vi "Tips.vi"() -> ()   [LabVIEW 2022 SP3]
panel:
  out "Numeric":i32
  out "x+y":dbl
  in  "y":dbl
  in  "x":dbl
  # "Ctrl + B 删除断线\nCtrl + R 运行程序\nCtrl+ E  更换面板"
  # "This is commit!"
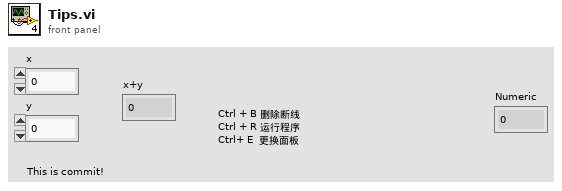
[diagram p1: front panel]
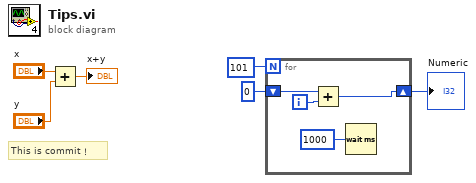
[diagram p0: block diagram]
diagram:
  # "This is commit！"
  n1 = Add(x="x", y="y") -> (x+y=→"x+y":dbl)
  n2 = for {
    N: 101 -> [_]
    shift-right: [w10] -> w1
    shift-left: 0 -> [w9]
    i -> [w8]
    n3 = Add(x=w9, y=w8) -> (x+y=w10:i32)
    n4 = Wait (ms)(milliseconds to wait=u32 1000) -> ()  [unwired: 1 out]
  }
  "Numeric" <- w1
